vi "Recipe Label Changed.vi"(8 "error in (no error)":errorcluster, 9 "New Label":string, 10 "Old Label":string, 11 "Main Window in":refnum<class "Main Window.lvclass">) -> (0 "error out":errorcluster, 3 "Main Window out":refnum<class "Main Window.lvclass">)   [LabVIEW 2021, in "Recipe.lvlib" / "Main Window.lvclass"]
uses:
  Main Window.lvclass
  Main Window.lvclass/Main Window.ctl
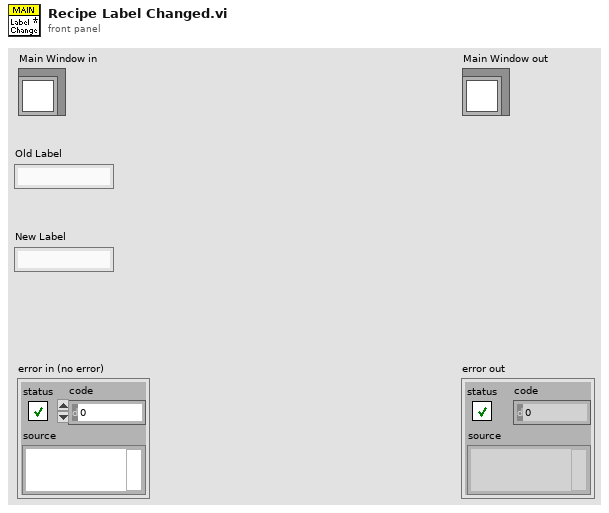
[diagram p1: front panel]
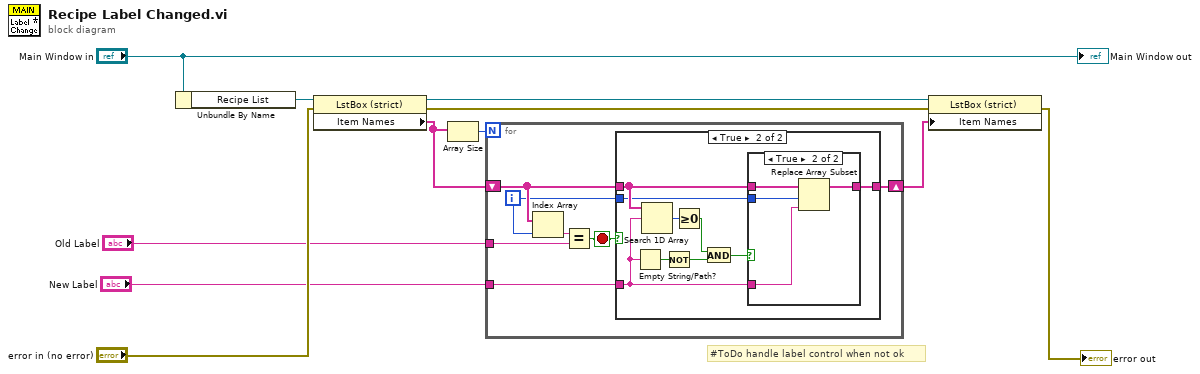
[diagram p0: block diagram]
diagram:
  # "#ToDo handle label control when not ok"
  n1 = Unbundle By Name("Main Window in") -> ("Recipe List"=w9:refnum<vi>)
  n2 = property class="LstBox (strict)"(reference=w9, error in="error in (no error)") -> (reference out=w8:refnum<vi>, error out=w7:errorcluster, "Item Names"=w1:string[])
  n3 = Array Size(array=w1) -> (size(s)=w2:i32)
  n4 = for {
    N: w2 -> [_]
    tunnel: "Old Label" -> [w18]
    tunnel: "New Label" -> [w17]
    shift-right: [w16] -> w3
    shift-left: w1 -> [w15]
    i -> [w12]
    stop <- w13 stop-if-true
    n5 = Index Array(array=w15, index=w12) -> (element=w14:string)
    n6 = Equal?(x=w14, y=w18) -> (x = y?=w13:bool)
    n7 = case shown="True" w13 {
      tunnel: w17 -> [_ w21]
      tunnel: [w19 w23] -> w16
      tunnel: w15 -> [w19 w24]
      tunnel: w12 -> [_ w20]
      frame False {
      }
      frame True {
        n8 = Empty String/Path?(string/path=w21) -> (empty?=w28:bool)
        n9 = Search 1D Array(1D array=w24, element=w21) -> (index of element=w27:i32)  [unwired: 1 in]
        n10 = Not(x=w28) -> (.not. x?=w25:bool)
        n11 = Greater Or Equal To 0?(x=w27) -> (x >= 0?=w26:bool)
        n12 = And(x=w26, y=w25) -> (x .and. y?=w22:bool)
        n13 = case shown="True" w22 {
          tunnel: w24 -> [w29 w33]
          tunnel: [w29 w32] -> w23
          tunnel: w21 -> [_ w31]
          tunnel: w20 -> [_ w30]
          frame False {
            # "#ToDo Message"
          }
          frame True {
            n14 = Replace Array Subset(array=w33, new element=w31, index=w30) -> (w32:string[])
          }
        }
      }
    }
  }
  n15 = property class="LstBox (strict)"(reference=w8, error in=w7, "Item Names"=w3) -> (error out=→"error out":errorcluster)  [unwired: 1 out]
  "Main Window out" <- "Main Window in"
